vi "Test_AI.vi"() -> ()   [LabVIEW 2023]
uses:
  Driver_AI_AO/Driver_AI_AO.lvclass
panel:
  in  "stop":bool
  out "Value":i32
  in  "Input":T1
  out "STATUS":string
  out "error out":errorcluster
  out "Error":string
  in  "PIN":i8
  in  "error in (no error)":errorcluster
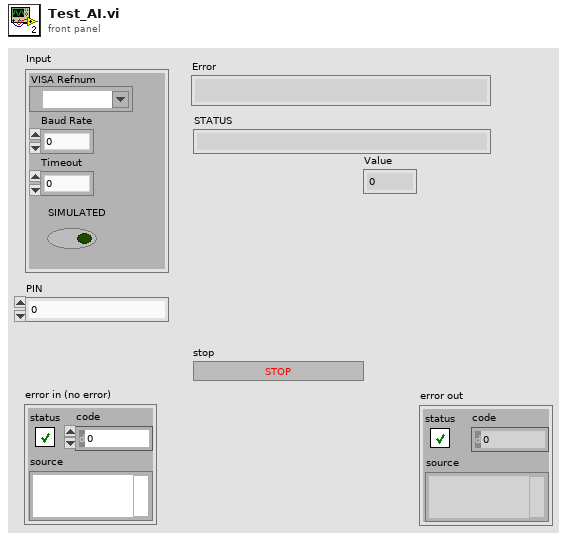
[diagram p1: front panel]
types:
  T1 = cluster{"VISA Refnum":refnum<visa-resource-name>, "Baud Rate":u32, "Timeout":u32, "SIMULATED":bool}
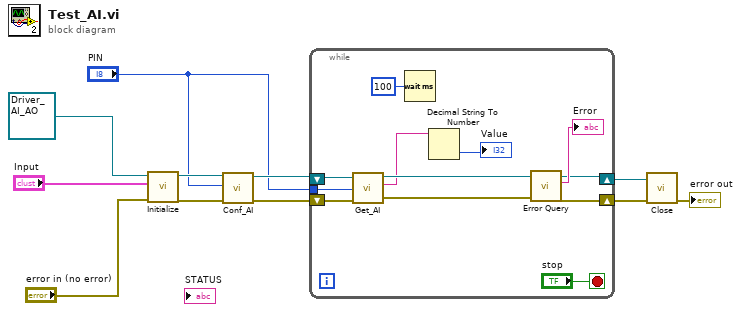
[diagram p0: block diagram]
diagram:
  n1 = call-dynamic "Initialize.vi"("error in (no error)"="error in (no error)", "Input"="Input", "Driver in"=refnum<class "Driver_AI_AO.lvclass"> refnum ("Driver_AI_AO.lvlib:Driver_AI_AO.lvclass")) -> ("error out"=w6:errorcluster, "Driver out"=w7:refnum<class "Driver_AI_AO.lvclass">)  [unwired: 7 in]
  n2 = call-dynamic "Conf_AI.vi"("error in (no error)"=w6, "PIN Number"="PIN", "Driver_AI_AO in"=w7) -> ("error out"=w5:errorcluster, "Driver_AI_AO out"=w4:refnum<class "Driver_AI_AO.lvclass">)  [unwired: 7 in]
  n3 = while {
    tunnel: "PIN" -> [w16]
    shift-right: [w17] -> w2
    shift-left: w5 -> [w22]
    shift-right: [w18] -> w3
    shift-left: w4 -> [w19]
    stop <- "stop" stop-if-true
    n4 = call-dynamic "Get_AI.vi"("error in (no error)"=w22, "PIN Number"=w16, "Driver_AI_AO in"=w19) -> ("error out"=w21:errorcluster, "STATUS"=w13:string, "Driver_AI_AO out"=w20:refnum<class "Driver_AI_AO.lvclass">)  [unwired: 6 in]
    n5 = Wait (ms)(milliseconds to wait=u32 100) -> ()  [unwired: 1 out]
    n6 = Decimal String To Number(string=w13) -> (number=→"Value":i32)  [unwired: 2 in, 1 out]
    n7 = call-dynamic "Error Query.vi"("error in (no error)"=w21, "Driver in"=w20) -> ("error out"=w17:errorcluster, "read buffer"=→"Error":string, "Driver out"=w18:refnum<class "Driver_AI_AO.lvclass">)  [unwired: 7 in]
  }
  n8 = call-dynamic "Close.vi"("error in (no error)"=w2, "Driver in"=w3) -> ("error out"=→"error out":errorcluster)  [unwired: 8 in, 1 out]
